vi "Vision Processing.vi"(4 "error in (no error)":errorcluster, 7 "Image Size":T1=enum."320x240") -> ()   [LabVIEW 2014]
doc: "This VI runs in parallel to other tasks. It gets images from the camera, processes them for color or shape and use that information to affect robot behavior."
uses:
  <vilib>/Rock Robotics/WPI/Camera/WPI_CameraImageSize.ctl
  <vilib>/Rock Robotics/WPI/Camera/WPI_CameraWhite Balance Values.ctl
  <vilib>/Rock Robotics/WPI/Camera/WPI_CameraExposure Values.ctl
  <vilib>/Rock Robotics/WPI/Camera/WPI_CameraFrameRate.ctl
  Robot Global Data.vi
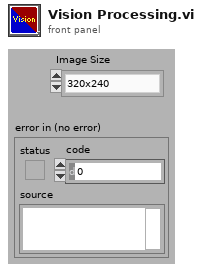
[diagram p1: front panel]
types:
  T1 = typedef "WPI_CameraImageSize.ctl" = enum16{"640x480", "320x240", "160x120", "Custom"}
  T2 = typedef "WPI_CameraFrameRate.ctl" = u32
  T3 = typedef "WPI_CameraExposure Values.ctl" = enum16{"Auto", "Flicker-free 50 Hz", "Flicker-free 60 Hz", "Hold current", "Custom"}
  T4 = typedef "WPI_CameraWhite Balance Values.ctl" = enum16{"Auto", "Fixed indoor", "Fixed outdoor 1", "Fixed outdoor 2", "Fixed fluorescent 1", "Fixed fluorescent 2", "Hold current", "Custom"}
  T5 = typedef "Image Type" = u32
  T6 = typedef "WPI_CameraDevRef.ctl" = cluster{"Camera Address":string, "CameraStatus":errorcluster}
  T7 = typedef "IMAQ Image.ctl" = refnum<image>
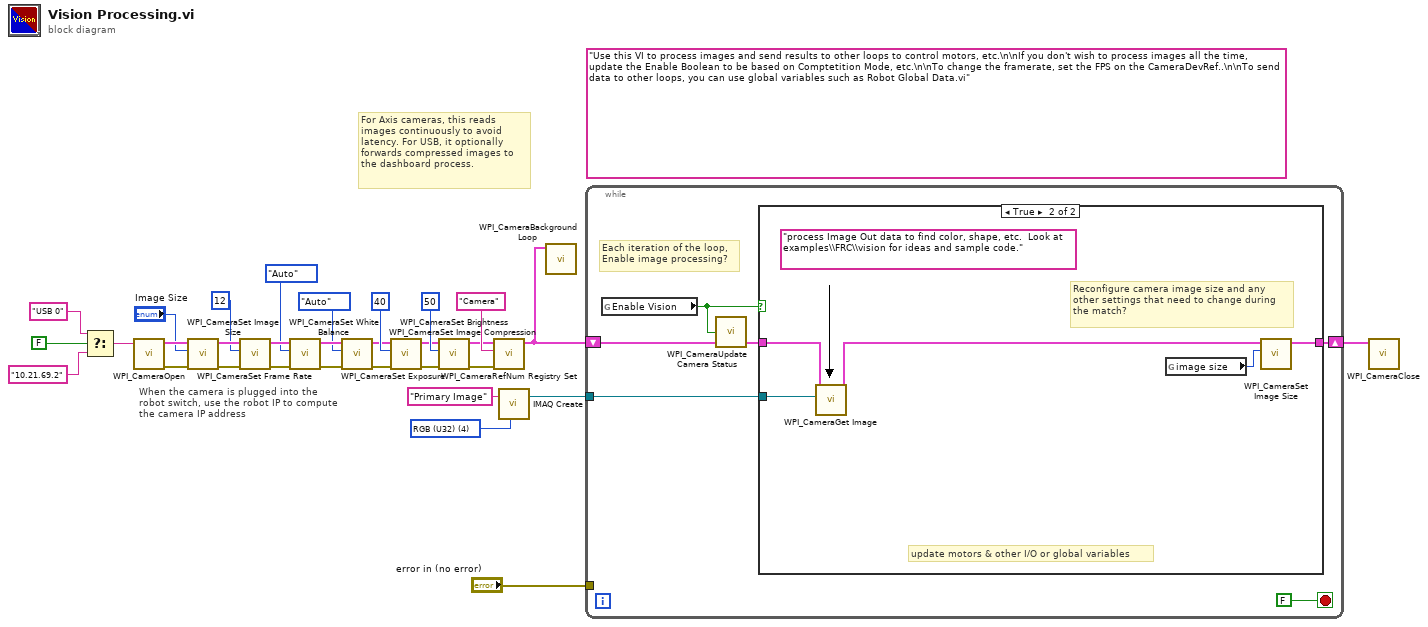
[diagram p0: block diagram]
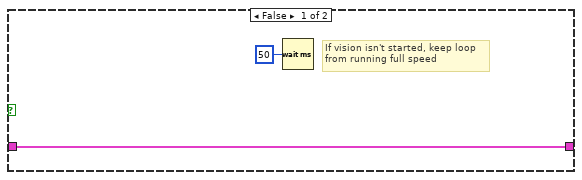
[diagram p2: hidden frame]
diagram:
  (unwired) "Use this VI to process images and send results to other loops to control motors, etc.\n\nIf you don't wish to process images all the time, update the Enable Boolean to be based on Comptetition Mode, etc.\n\nTo change the framerate, set the FPS on the CameraDevRef..\n\nTo send data to other loops, you can use global variables such as Robot Global Data.vi"
  w31 = T5 4 items=["Grayscale (U8)", "Grayscale (I16)", "Grayscale (SGL)", "Complex (CSG)", "RGB (U32)", "HSL (U32)", "RGB (U64)"] ("Image Type")
  # "When the camera is plugged into the\nrobot switch, use the robot IP to compute\nthe camera IP address"
  # "For Axis cameras, this reads\nimages continuously to avoid\nlatency. For USB, it optionally\nforwards compressed images to\nthe dashboard process."
  n1 = Select(t="USB 0" ("format string"), s=FALSE ("dot notation? (F)"), f="10.21.69.2" ("format string")) -> (s? t:f=w2:string)
  n2 = call <vilib>:"WPI_CameraOpen.vi"("Camera Address"=w2) -> ("error out"=w19:errorcluster, "CameraDevRef"=w20:T6)  [unwired: 1 in, 8 out]
  n3 = call <vilib>:"WPI_CameraSet Image Size.vi"("error in (no error)"=w19, "Image Size"="Image Size", "CameraDevRef"=w20) -> ("error out"=w18:errorcluster, "CameraDevRef Out"=w21:T6)  [unwired: 1 in, 6 out]
  n4 = call <vilib>:"WPI_CameraSet Frame Rate.vi"("error in (no error)"=w18, "Frame Rate (fps)"=T2 12, "CameraDevRef"=w21) -> ("error out"=w17:errorcluster, "CameraDevRef Out"=w23:T6)  [unwired: 7 out]
  n5 = call <vilib>:"WPI_CameraSet White Balance.vi"("error in (no error)"=w17, "White Balance"=WPI_CameraWhite_Balance_Values."Auto", "CameraDevRef"=w23) -> ("error out"=w16:errorcluster, "CameraDevRef Out"=w22:T6)  [unwired: 1 in, 6 out]
  n6 = call <vilib>:"WPI_CameraSet Exposure.vi"("error in (no error)"=w16, "Exposure"=WPI_CameraExposure_Values."Auto", "CameraDevRef"=w22) -> ("error out"=w15:errorcluster, "CameraDevRef Out"=w25:T6)  [unwired: 1 in, 6 out]
  n7 = call <vilib>:"WPI_CameraSet Image Compression.vi"("error in (no error)"=w15, "Compression"=40, "CameraDevRef"=w25) -> ("error out"=w14:errorcluster, "CameraDevRef Out"=w24:T6)  [unwired: 7 out]
  n8 = call <vilib>:"WPI_CameraSet Brightness.vi"("error in (no error)"=w14, "Brightness"=50, "CameraDevRef"=w24) -> ("error out"=w12:errorcluster, "CameraDevRef Out"=w13:T6)  [unwired: 7 out]
  n9 = call <vilib>:"WPI_CameraRefNum Registry Set.vi"("error in (no error)"=w12, "refnum name"="Camera", "CameraDevRef"=w13) -> ("CameraDevRef"=w8:T6)  [unwired: 8 out]
  n10 = call "IMAQ Create"("Image Name"="Primary Image", "Image Type"=w31) -> ("New Image"=w29:T7)  [unwired: 2 in, 2 out]
  n11 = call <vilib>:"WPI_CameraBackground Loop.vi"("CameraDevRef"=w8) -> ()  [unwired: 11 in]
  n12 = while {
    shift-right: [w36] -> w6
    shift-left: w8 -> [w34]
    tunnel: w29 -> [w35]
    tunnel: "error in (no error)" -> [_]
    stop <- FALSE stop-if-true
    # "Each iteration of the loop,\nEnable image processing?"
    n13 = global read "Robot Global Data.vi" "Enable Vision"() -> (w32:bool)
    n14 = call <vilib>:"WPI_CameraUpdate Camera Status.vi"("CameraDevRef In"=w34, "Enable Vision"=w32) -> ("CameraDevRef Out"=w33:T6)  [unwired: 3 in]
    n15 = case shown="True" w32 {
      tunnel: w35 -> [_ w43]
      tunnel: [w39 w44] -> w36
      tunnel: w33 -> [w39 w41]
      frame False {
        # "If vision isn't started, keep loop\nfrom running full speed"
        n16 = Wait (ms)(milliseconds to wait=u32 50) -> ()  [unwired: 1 out]
      }
      frame True {
        (unwired) "process Image Out data to find color, shape, etc.  Look at examples\\FRC\\vision for ideas and sample code."
        # "update motors & other I/O or global variables"
        # "Reconfigure camera image size and any\nother settings that need to change during\nthe match?"
        n17 = call <vilib>:"WPI_CameraGet Image.vi"("Image"=w43, "CameraDevRef"=w41) -> ("CameraDevRef Out"=w40:T6)  [unwired: 1 in, 8 out]
        n18 = global read "Robot Global Data.vi" "image size"() -> (w42:T1)
        n19 = call <vilib>:"WPI_CameraSet Image Size.vi"("Image Size"=w42, "CameraDevRef"=w40) -> ("CameraDevRef Out"=w44:T6)  [unwired: 2 in, 7 out]
      }
    }
  }
  n20 = call <vilib>:"WPI_CameraClose.vi"("CameraDevRef"=w6) -> ()  [unwired: 1 in, 10 out]
